vi "choosePlayVSS.vi"(8 "error in (no error)":errorcluster, 10 "queue":T1(array[ring]), 11 "Game in":refnum<class "Game.lvclass">) -> (0 "error out":errorcluster, 2 "output queue":T1(array[ring]), 3 "Game out":refnum<class "Game.lvclass">)   [LabVIEW 2020, in "Game.lvclass"]
uses:
  Game.lvclass
  Command.ctl
  Game.lvclass/Game.ctl
  HaltPlay_class/HaltPlay.lvclass
  TimeoutPlay_class/TimeoutPlay.lvclass
  NormalGamePlayVSS_class/NormalGamePlayVSS.lvclass
  KickPenaltyAllyPlayVSS_class/KickPenaltyAllyPlayVSS.lvclass
  PenaltyEnemyPlayVSS_class/PenaltyEnemyPlayVSS.lvclass
  BallChallengePlayVSS_class/BallChallengePlayVSS.lvclass
  PreparePenaltyAllyPlayVSS_class/PreparePenaltyAllyPlayVSS.lvclass
  DeadBallPlayVSS_class/DeadBallPlayVSS.lvclass
  PreparePenaltyEnemyPlayVSS_class/PreparePenaltyEnemyPlayVSS.lvclass
  PrepareKickoffAllyPlayVSS_class/PrepareKickoffAllyPlayVSS.lvclass
  PrepareKickoffEnemyPlayVSS_class/PrepareKickoffEnemyPlayVSS.lvclass
  StopPlayVSS_class/StopPlayVSS.lvclass
  PrepareGoalKickAllyPlayVSS_class/PrepareGoalKickAllyPlayVSS.lvclass
  PrepareGoalKickEnemyPlayVSS_class/PrepareGoalKickEnemyPlayVSS.lvclass
  KickoffEnemyPlayVSS_class/KickoffEnemyPlayVSS.lvclass
  KickoffAllyPlayVSS_class/KickoffAllyPlayVSS.lvclass
  GoalKickAllyPlayVSS_class/GoalKickAllyPlayVSS.lvclass
  GoalKickEnemyPlayVSS_class/GoalKickEnemyPlayVSS.lvclass
  PrepareFreeBallPlayVSS_class/PrepareFreeBallPlayVSS.lvclass
  FreeBallPlayVSS_class/FreeBallPlayVSS.lvclass
  Read KeeperTeam.vi
  Read Referee.vi
  Read AllyRef.vi
  Write AllyRef.vi
  Write KeeperTeam.vi
  Ally_class/Ally.lvclass
  C:/Users/lucio/Desktop/Horie/ROBOIME/VSS_AI/Team_class/Team.lvclass
  Referee_class/Referee.lvclass
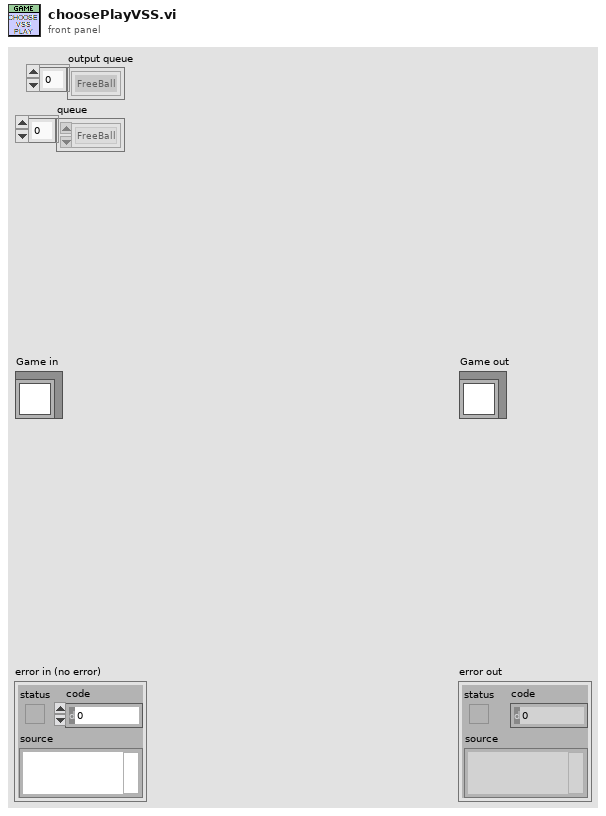
[diagram p1: front panel]
types:
  T1 = enum16{"FreeBall", "PrepareFreeBall", "GoalKickEnemy", "GoalKickAlly", "KickoffAlly", "KickoffEnemy", "PrepareGoalKickEnemy", "PrepareGoalKickAlly", "Stop", "PrepareKickoffEnemy", "PrepareKickoffAlly", "PreparePenaltyEnemy", "Timeout", "DeadBall", "NormalGame", "KickPenaltyAlly", "PenaltyEnemy", "BallChallenge", "PreparePenaltyAlly", "Halt"}[]
  T2 = typedef "Command.ctl" = enum16{"AUTO", "GAME_ON", "STOP", "HALT", "KICKOFF_ALLY", "KICKOFF_ENEMY", "FREE_BALL", "GOAL_KICK_ENEMY", "GOAL_KICK_ALLY", "PENALTY_KICK_ENEMY", "PENALTY_KICK_ALLY", "FREE_KICK"}
  T3 = enum16{"FreeBall", "PrepareFreeBall", "GoalKickEnemy", "GoalKickAlly", "KickoffAlly", "KickoffEnemy", "PrepareGoalKickEnemy", "PrepareGoalKickAlly", "Stop", "PrepareKickoffEnemy", "PrepareKickoffAlly", "PreparePenaltyEnemy", "Timeout", "DeadBall", "NormalGame", "KickPenaltyAlly", "PenaltyEnemy", "BallChallenge", "PreparePenaltyAlly", "Halt"}
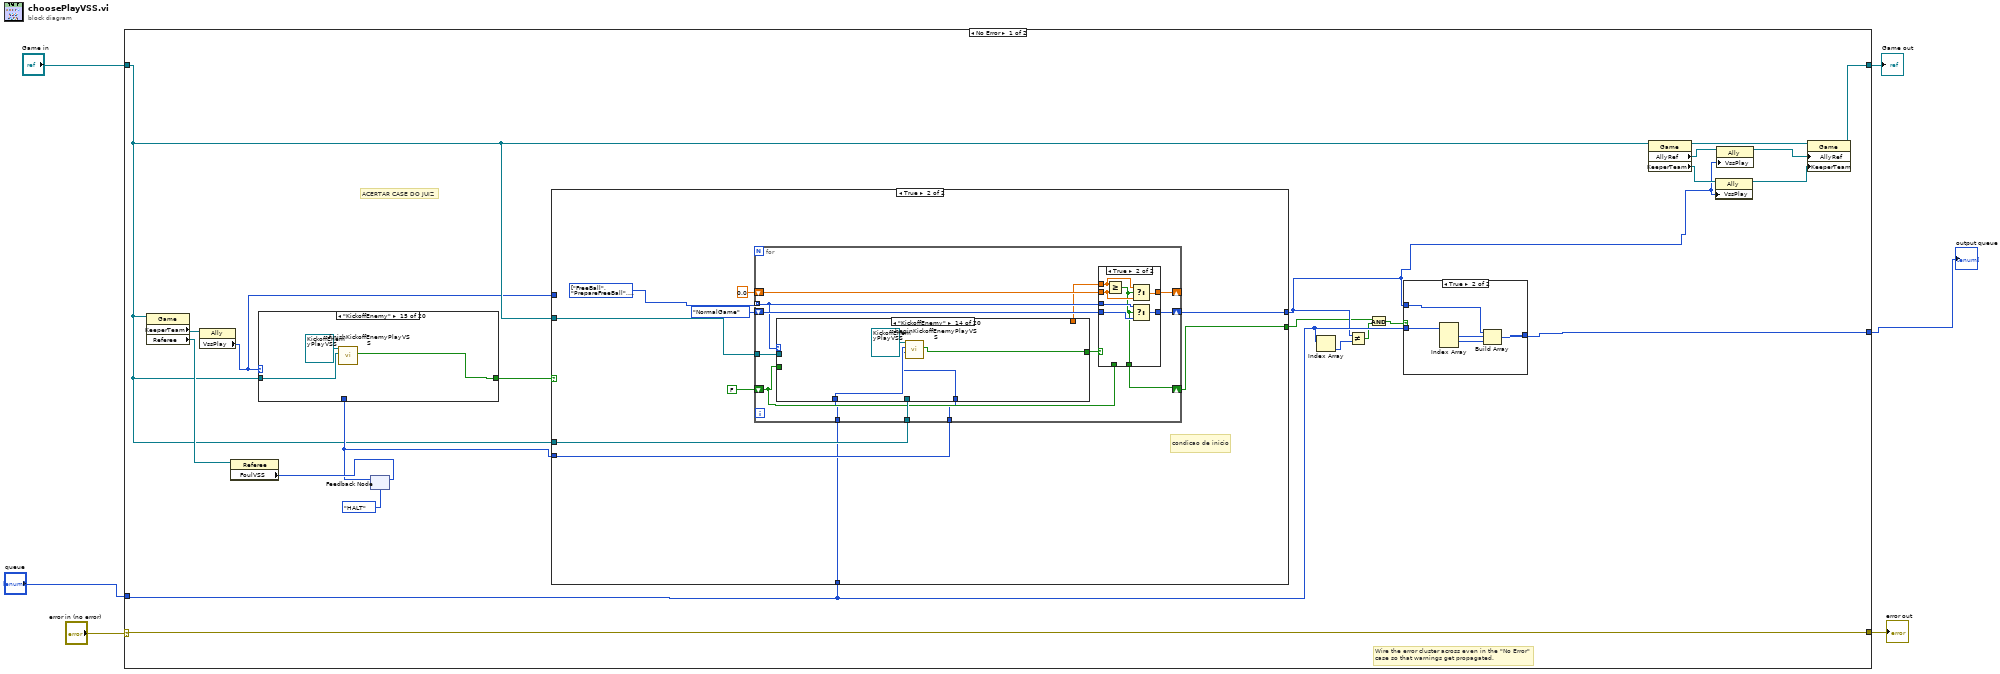
[diagram p0: block diagram]
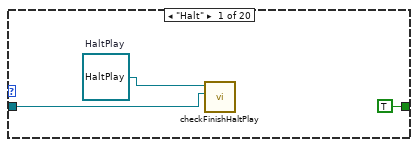
[diagram p3: hidden frame]
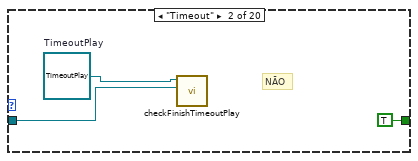
[diagram p4: hidden frame]
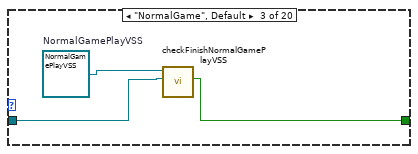
[diagram p5: hidden frame]
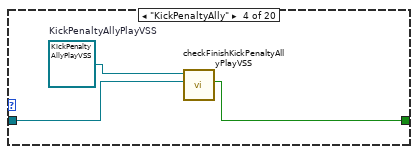
[diagram p6: hidden frame]
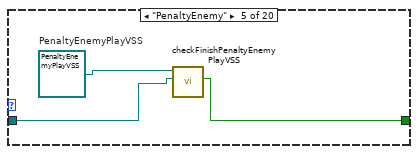
[diagram p7: hidden frame]
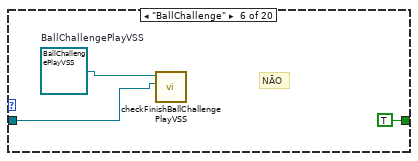
[diagram p8: hidden frame]
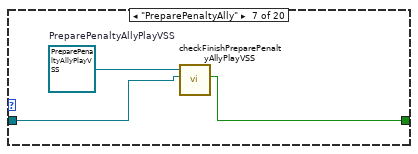
[diagram p9: hidden frame]
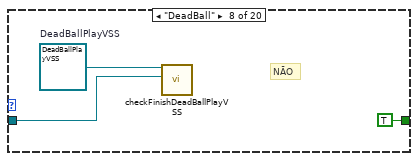
[diagram p10: hidden frame]
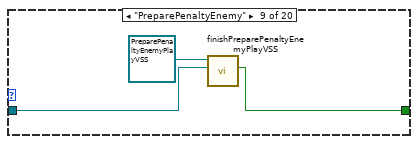
[diagram p11: hidden frame]
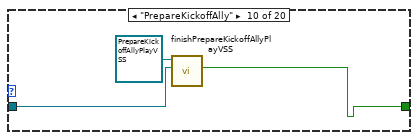
[diagram p12: hidden frame]
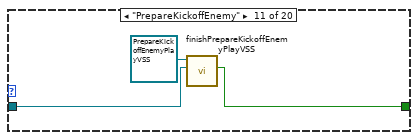
[diagram p13: hidden frame]
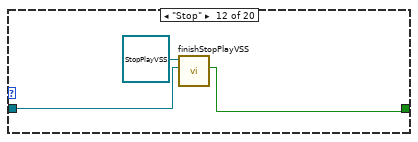
[diagram p14: hidden frame]
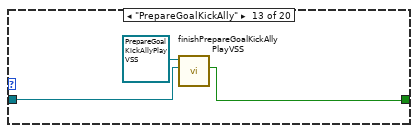
[diagram p15: hidden frame]
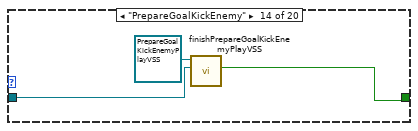
[diagram p16: hidden frame]
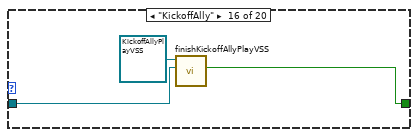
[diagram p17: hidden frame]
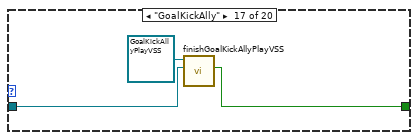
[diagram p18: hidden frame]
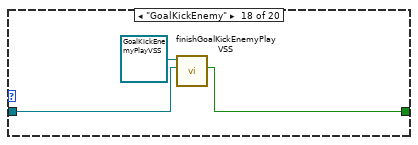
[diagram p19: hidden frame]
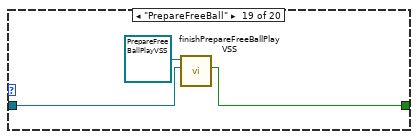
[diagram p20: hidden frame]
diagram:
  n1 = case shown="No Error" "error in (no error)" {
    selector: "error in (no error)" -> [w28 w199]
    tunnel: [w28 w199] -> w5
    tunnel: [w26 w198] -> w3
    tunnel: "Game in" -> [w17 w198]
    tunnel: "queue" -> [w12 _]
    tunnel: [w14 _] -> w1
    frame No Error {
      # "ACERTAR CASE DO JUIZ"
      # "Wire the error cluster across even in the \"No Error\"\ncase so that warnings get propagated."
      n2 = property class="Game"(reference=w17) -> ("KeeperTeam"=w16:refnum<class "Ally.lvclass">, "Referee"=w20:refnum<class "Referee.lvclass">)  [unwired: 1 in, 2 out]
      n3 = property class="Ally"(reference=w16) -> ("VssPlay"=w15:T3)  [unwired: 1 in, 2 out]
      n4 = property class="Referee"(reference=w20) -> ("FoulVSS"=w19:T2)  [unwired: 1 in, 2 out]
      n5 = feedback-in #1(w19) -> ()
      n6 = feedback #1(Command."HALT" ("FoulVSS")) -> (w18:T2)
      n7 = case shown="\"KickoffEnemy\"" w15 {
        tunnel: [TRUE ("result") TRUE ("Boolean") w41 w44 w47 TRUE ("Boolean") w53 TRUE ("Boolean") w59 w62 w65 w68 w71 w74 w77 w80 w83 w86 w89 w92] -> w25
        tunnel: w17 -> [w36 w39 w42 w45 w48 w51 w54 w58 w60 w63 w66 w69 w72 w75 w78 w81 w84 w87 w90 w93]
        tunnel: w18 -> [_ _ _ _ _ _ _ _ _ _ _ _ _ _ _ _ _ _ _ _]
        frame "Halt" {
          w37 = refnum<class "HaltPlay.lvclass"> refnum  # HaltPlay
          n8 = call "checkFinishHaltPlay.vi"("Game"=w36, "HaltPlay in"=w37) -> ()  [unwired: 7 in, 3 out]
        }
        frame "Timeout" {
          w40 = refnum<class "TimeoutPlay.lvclass"> refnum  # TimeoutPlay
          # "NÃO"
          n9 = call "checkFinishTimeoutPlay.vi"("Game"=w39, "TimeoutPlay in"=w40) -> ()  [unwired: 7 in, 3 out]
        }
        frame "NormalGame", Default {
          w43 = refnum<class "NormalGamePlayVSS.lvclass"> refnum  # NormalGamePlayVSS
          n10 = call "checkFinishNormalGamePlayVSS.vi"("Game in"=w42, "NormalGamePlayVSS in"=w43) -> ("Boolean"=w41:bool)  [unwired: 7 in, 2 out]
        }
        frame "KickPenaltyAlly" {
          w46 = refnum<class "KickPenaltyAllyPlayVSS.lvclass"> refnum  # KickPenaltyAllyPlayVSS
          n11 = call "checkFinishKickPenaltyAllyPlayVSS.vi"("Game in"=w45, "KickPenaltyAllyPlayVSS in"=w46) -> ("result"=w44:bool)  [unwired: 7 in, 2 out]
        }
        frame "PenaltyEnemy" {
          w49 = refnum<class "PenaltyEnemyPlayVSS.lvclass"> refnum  # PenaltyEnemyPlayVSS
          n12 = call "checkFinishPenaltyEnemyPlayVSS.vi"("Game in"=w48, "PenaltyEnemyPlayVSS in"=w49) -> ("result"=w47:bool)  [unwired: 7 in, 2 out]
        }
        frame "BallChallenge" {
          w52 = refnum<class "BallChallengePlayVSS.lvclass"> refnum  # BallChallengePlayVSS
          # "NÃO"
          n13 = call "checkFinishBallChallengePlayVSS.vi"("Game in"=w51, "BallChallengePlayVSS in"=w52) -> ()  [unwired: 7 in, 3 out]
        }
        frame "PreparePenaltyAlly" {
          w55 = refnum<class "PreparePenaltyAllyPlayVSS.lvclass"> refnum  # PreparePenaltyAllyPlayVSS
          n14 = call "checkFinishPreparePenaltyAllyPlayVSS.vi"("Game"=w54, "PreparePenaltyAllyPlayVSS in"=w55) -> ("Boolean"=w53:bool)  [unwired: 7 in, 2 out]
        }
        frame "DeadBall" {
          w57 = refnum<class "DeadBallPlayVSS.lvclass"> refnum  # DeadBallPlayVSS
          # "NÃO"
          n15 = call "checkFinishDeadBallPlayVSS.vi"("Game"=w58, "DeadBallPlayVSS in"=w57) -> ()  [unwired: 7 in, 3 out]
        }
        frame "PreparePenaltyEnemy" {
          n16 = call "finishPreparePenaltyEnemyPlayVSS.vi"("Game in"=w60, "PreparePenaltyEnemyPlayVSS in"=refnum<class "PreparePenaltyEnemyPlayVSS.lvclass"> refnum) -> ("Boolean"=w59:bool)  [unwired: 7 in, 2 out]
        }
        frame "PrepareKickoffAlly" {
          n17 = call "finishPrepareKickoffAllyPlayVSS.vi"("Game in"=w63, "PrepareKickoffAllyPlayVSS in"=refnum<class "PrepareKickoffAllyPlayVSS.lvclass"> refnum) -> ("Boolean"=w62:bool)  [unwired: 7 in, 2 out]
        }
        frame "PrepareKickoffEnemy" {
          n18 = call "finishPrepareKickoffEnemyPlayVSS.vi"("Game in"=w66, "PrepareKickoffEnemyPlayVSS in"=refnum<class "PrepareKickoffEnemyPlayVSS.lvclass"> refnum) -> ("Boolean"=w65:bool)  [unwired: 7 in, 2 out]
        }
        frame "Stop" {
          n19 = call "finishStopPlayVSS.vi"("Game in"=w69, "StopPlayVSS in"=refnum<class "StopPlayVSS.lvclass"> refnum) -> ("Boolean"=w68:bool)  [unwired: 7 in, 2 out]
        }
        frame "PrepareGoalKickAlly" {
          n20 = call "finishPrepareGoalKickAllyPlayVSS.vi"("Game in 2"=w72, "PrepareGoalKickAllyPlayVSS in"=refnum<class "PrepareGoalKickAllyPlayVSS.lvclass"> refnum) -> ("Boolean"=w71:bool)  [unwired: 7 in, 2 out]
        }
        frame "PrepareGoalKickEnemy" {
          n21 = call "finishPrepareGoalKickEnemyPlayVSS.vi"("Game in 2"=w75, "PrepareGoalKickEnemyPlayVSS in"=refnum<class "PrepareGoalKickEnemyPlayVSS.lvclass"> refnum) -> ("Boolean"=w74:bool)  [unwired: 7 in, 2 out]
        }
        frame "KickoffEnemy" {
          n22 = call "finishKickoffEnemyPlayVSS.vi"("Game in"=w78, "KickoffEnemyPlayVSS in"=refnum<class "KickoffEnemyPlayVSS.lvclass"> refnum) -> ("result"=w77:bool)  [unwired: 7 in, 2 out]
        }
        frame "KickoffAlly" {
          n23 = call "finishKickoffAllyPlayVSS.vi"("Game in"=w81, "KickoffAllyPlayVSS in"=refnum<class "KickoffAllyPlayVSS.lvclass"> refnum) -> ("result"=w80:bool)  [unwired: 7 in, 2 out]
        }
        frame "GoalKickAlly" {
          n24 = call "finishGoalKickAllyPlayVSS.vi"("Game in"=w84, "GoalKickAllyPlayVSS in"=refnum<class "GoalKickAllyPlayVSS.lvclass"> refnum) -> ("result"=w83:bool)  [unwired: 7 in, 2 out]
        }
        frame "GoalKickEnemy" {
          n25 = call "finishGoalKickEnemyPlayVSS.vi"("Game in"=w87, "GoalKickEnemyPlayVSS in"=refnum<class "GoalKickEnemyPlayVSS.lvclass"> refnum) -> ("result"=w86:bool)  [unwired: 7 in, 2 out]
        }
        frame "PrepareFreeBall" {
          n26 = call "finishPrepareFreeBallPlayVSS.vi"("Game in 2"=w90, "PrepareFreeBallPlayVSS in"=refnum<class "PrepareFreeBallPlayVSS.lvclass"> refnum) -> ("Boolean"=w89:bool)  [unwired: 7 in, 2 out]
        }
        frame "FreeBall" {
          n27 = call "finishFreeBallPlayVSS.vi"("Game in"=w93, "FreeBallPlayVSS in"=refnum<class "FreeBallPlayVSS.lvclass"> refnum) -> ("result"=w92:bool)  [unwired: 7 in, 2 out]
        }
      }
      n28 = case shown="True" w25 {
        tunnel: [w96 w105] -> w10
        tunnel: w15 -> [w96 _]
        tunnel: w17 -> [_ w104]
        tunnel: w18 -> [_ w102]
        tunnel: w17 -> [_ w101]
        tunnel: [FALSE w99] -> w8
        tunnel: w12 -> [_ w98]
        frame False {
        }
        frame True {
          w100 = T1 [enum."FreeBall", enum."PrepareFreeBall", enum."GoalKickEnemy", enum."GoalKickAlly", enum."KickoffAlly", enum."KickoffEnemy", enum."PrepareGoalKickEnemy", enum."PrepareGoalKickAlly", enum."Stop", enum."PrepareKickoffEnemy", enum."PrepareKickoffAlly", enum."PreparePenaltyEnemy", enum."Timeout", enum."DeadBall", enum."KickPenaltyAlly", enum."PenaltyEnemy", enum."BallChallenge", enum."PreparePenaltyAlly", enum."Halt", enum."NormalGame"] items=["FreeBall", "PrepareFreeBall", "GoalKickEnemy", "GoalKickAlly", "KickoffAlly", "KickoffEnemy", "PrepareGoalKickEnemy", "PrepareGoalKickAlly", "Stop", "PrepareKickoffEnemy", "PrepareKickoffAlly", "PreparePenaltyEnemy", "Timeout", "DeadBall", "NormalGame", "KickPenaltyAlly", "PenaltyEnemy", "BallChallenge", "PreparePenaltyAlly", "Halt"] ("VssPlay")
          # "condicao de inicio"
          n29 = for {
            tunnel: w100 -> [w115] mode=indexing
            shift-right: [w118] -> _
            shift-left: 0.0 -> [w117]
            shift-right: [w116] -> w105
            shift-left: T3."NormalGame" ("VssPlay") -> [w119]
            tunnel: w104 -> [w112]
            shift-right: [w111] -> w99
            shift-left: FALSE -> [w110]
            tunnel: w102 -> [w109]
            tunnel: w101 -> [w108]
            tunnel: w98 -> [w107]
            n30 = case shown="\"KickoffEnemy\"" w115 {
              tunnel: [w120 w124 FALSE ("Boolean") w132 FALSE ("Boolean") FALSE ("Boolean") w145 w150 w151 w154 w157 w160 w163 w167 w170 w173 w176 w179 w182 w185] -> w114
              tunnel: [0.0 0.0 0.0 0.0 0.0 0.0 0.0 0.0 _ _ _ _ _ _ _ _ _ _ _ _] -> w113
              tunnel: w112 -> [w122 _ _ _ _ _ _ _ _ w155 _ _ _ _ w171 w175 w177 w180 w183 _]
              tunnel: w110 -> [_ _ _ _ _ _ _ w149 _ _ _ _ _ _ _ _ _ _ _ _]
              tunnel: w109 -> [_ _ _ _ _ _ _ _ _ _ _ _ _ w166 _ _ _ _ _ _]
              tunnel: w108 -> [_ _ w130 _ w137 w141 w146 _ _ _ _ _ _ _ _ _ _ _ _ w186]
              tunnel: w107 -> [_ w125 _ w133 _ _ _ _ w152 _ w158 w161 w164 w168 _ _ _ _ _ _]
              frame "Halt" {
                w123 = refnum<class "HaltPlay.lvclass"> refnum  # HaltPlay
                # "NÃO"
                n31 = call "checkBeginHaltPlay.vi"("Game"=w122, "HaltPlay in"=w123) -> ("Boolean"=w120:bool)  [unwired: 7 in, 2 out]
              }
              frame "KickPenaltyAlly" {
                w126 = refnum<class "KickPenaltyAllyPlayVSS.lvclass"> refnum  # KickPenaltyAllyPlayVSS
                n32 = call "checkBeginKickPenaltyAllyPlayVSS.vi"("queue 2"=w125, "KickPenaltyAllyPlayVSS in"=w126) -> ("logical AND"=w124:bool)  [unwired: 7 in, 2 out]
              }
              frame "Timeout" {
                w131 = refnum<class "TimeoutPlay.lvclass"> refnum  # TimeoutPlay
                # "NÃO"
                n33 = call "checkBeginTimeoutPlay.vi"("Game"=w130, "TimeoutPlay in"=w131) -> ()  [unwired: 7 in, 3 out]
              }
              frame "PenaltyEnemy" {
                n34 = call "checkBeginPenaltyEnemyPlayVSS.vi"("queue 2"=w133, "PenaltyEnemyPlayVSS in"=refnum<class "PenaltyEnemyPlayVSS.lvclass"> refnum) -> ("logical AND"=w132:bool)  [unwired: 7 in, 2 out]
              }
              frame "BallChallenge" {
                # "NÃO"
                n35 = call "checkBeginBallChallengePlayVSS.vi"("Game"=w137, "BallChallengePlayVSS in"=refnum<class "BallChallengePlayVSS.lvclass"> refnum) -> ()  [unwired: 7 in, 3 out]
              }
              frame "DeadBall" {
                # "NÃO"
                n36 = call "checkBeginDeadBallPlayVSS.vi"("Game"=w141, "DeadBallPlayVSS in"=refnum<class "DeadBallPlayVSS.lvclass"> refnum) -> ()  [unwired: 7 in, 3 out]
              }
              frame "PreparePenaltyAlly" {
                w147 = refnum<class "PreparePenaltyAllyPlayVSS.lvclass"> refnum  # PreparePenaltyAllyPlayVSS
                n37 = call "checkBeginPreparePenaltyAllyPlayVSS.vi"("Game in"=w146, "PreparePenaltyAllyPlayVSS in"=w147) -> ("Boolean"=w145:bool)  [unwired: 7 in, 2 out]
              }
              frame "NormalGame", Default {
                n38 = Not(x=w149) -> (.not. x?=w150:bool)
              }
              frame "FreeBall" {
                n39 = call "beginFreeBallPlayVSS.vi"("queue 2"=w152, "FreeBallPlayVSS in"=refnum<class "FreeBallPlayVSS.lvclass"> refnum) -> ("logical AND"=w151:bool)  [unwired: 7 in, 2 out]
              }
              frame "PrepareFreeBall" {
                n40 = call "beginPrepareFreeBallPlayVSS.vi"("Game in"=w155, "PrepareFreeBallPlayVSS in"=refnum<class "PrepareFreeBallPlayVSS.lvclass"> refnum) -> ("Boolean"=w154:bool)  [unwired: 7 in, 2 out]
              }
              frame "GoalKickEnemy" {
                n41 = call "beginGoalKickEnemyPlayVSS.vi"("queue 2"=w158, "GoalKickEnemyPlayVSS in"=refnum<class "GoalKickEnemyPlayVSS.lvclass"> refnum) -> ("logical AND"=w157:bool)  [unwired: 7 in, 2 out]
              }
              frame "GoalKickAlly" {
                n42 = call "beginGoalKickAllyPlayVSS.vi"("queue 2"=w161, "GoalKickAllyPlayVSS in"=refnum<class "GoalKickAllyPlayVSS.lvclass"> refnum) -> ("logical AND"=w160:bool)  [unwired: 7 in, 2 out]
              }
              frame "KickoffAlly" {
                n43 = call "beginKickoffAllyPlayVSS.vi"("queue 2"=w164, "KickoffAllyPlayVSS in"=refnum<class "KickoffAllyPlayVSS.lvclass"> refnum) -> ("logical AND"=w163:bool)  [unwired: 7 in, 2 out]
              }
              frame "KickoffEnemy" {
                n44 = call "beginKickoffEnemyPlayVSS.vi"("FoulVSS"=w166, "queue 2"=w168, "KickoffEnemyPlayVSS in"=refnum<class "KickoffEnemyPlayVSS.lvclass"> refnum) -> ("logical AND"=w167:bool)  [unwired: 6 in, 2 out]
              }
              frame "PrepareGoalKickEnemy" {
                n45 = call "beginPrepareGoalKickEnemyPlayVSS.vi"("Game in"=w171, "PrepareGoalKickEnemyPlayVSS in"=refnum<class "PrepareGoalKickEnemyPlayVSS.lvclass"> refnum) -> ("Boolean"=w170:bool)  [unwired: 7 in, 2 out]
              }
              frame "PrepareGoalKickAlly" {
                n46 = call "beginPrepareGoalKickAllyPlayVSS.vi"("Game in"=w175, "PrepareGoalKickAllyPlayVSS in"=refnum<class "PrepareGoalKickAllyPlayVSS.lvclass"> refnum) -> ("Boolean"=w173:bool)  [unwired: 7 in, 2 out]
              }
              frame "Stop" {
                n47 = call "beginStopPlayVSS.vi"("Game in"=w177, "StopPlayVSS in"=refnum<class "StopPlayVSS.lvclass"> refnum) -> ("Boolean"=w176:bool)  [unwired: 7 in, 2 out]
              }
              frame "PrepareKickoffEnemy" {
                n48 = call "beginPrepareKickoffEnemyPlayVSS.vi"("Game in"=w180, "PrepareKickoffEnemyPlayVSS in"=refnum<class "PrepareKickoffEnemyPlayVSS.lvclass"> refnum) -> ("Boolean"=w179:bool)  [unwired: 7 in, 2 out]
              }
              frame "PrepareKickoffAlly" {
                n49 = call "beginPrepareKickoffAllyPlayVSS.vi"("Game in"=w183, "PrepareKickoffAllyPlayVSS in"=refnum<class "PrepareKickoffAllyPlayVSS.lvclass"> refnum) -> ("Boolean"=w182:bool)  [unwired: 7 in, 2 out]
              }
              frame "PreparePenaltyEnemy" {
                n50 = call "beginPreparePenaltyEnemyPlayVSS.vi"("Game in"=w186, "PreparePenaltyEnemyPlayVSS in"=refnum<class "PreparePenaltyEnemyPlayVSS.lvclass"> refnum) -> ("Boolean"=w185:bool)  [unwired: 7 in, 2 out]
              }
            }
            n51 = case shown="True" w114 {
              tunnel: w119 -> [w189 w194]
              tunnel: [w190 w197] -> w118
              tunnel: w117 -> [w190 w193]
              tunnel: w115 -> [_ w195]
              tunnel: [w189 w196] -> w116
              tunnel: w113 -> [_ w192]
              tunnel: [w188 w191] -> w111
              tunnel: w110 -> [w188 _]
              frame False {
              }
              frame True {
                n52 = Greater Or Equal?(x=w192, y=w193) -> (x >= y?=w191:bool)
                n53 = Select(t=w192, s=w191, f=w193) -> (s? t:f=w197:dbl)
                n54 = Select(t=w195, s=w191, f=w194) -> (s? t:f=w196:T3)
              }
            }
          }
        }
      }
      n55 = Index Array(array=w12) -> (element=w11:T3)  [unwired: 1 in]
      n56 = Not Equal?(x=w10, y=w11) -> (x != y?=w9:bool)
      n57 = And(x=w8, y=w9) -> (x .and. y?=w7:bool)
      n58 = case shown="True" w7 {
        tunnel: w12 -> [w29 w34]
        tunnel: w10 -> [_ w33]
        tunnel: [w29 w30] -> w14
        frame False {
        }
        frame True {
          n59 = Index Array(array=w34) -> (element #1=w32:T3, element #2=w31:T3)  [unwired: 3 in, 1 out]
          n60 = Build Array(w33, w32, w31) -> (w30:T1)
        }
      }
      n61 = property class="Game"(reference=w17) -> (reference out=w27:refnum<class "Game.lvclass">, "AllyRef"=w22:refnum<class "Ally.lvclass">, "KeeperTeam"=w24:refnum<class "Ally.lvclass">)  [unwired: 1 in, 1 out]
      n62 = property class="Ally"(reference=w24, "VssPlay"=w10) -> (reference out=w23:refnum<class "Ally.lvclass">)  [unwired: 1 in, 1 out]
      n63 = property class="Ally"(reference=w22, "VssPlay"=w10) -> (reference out=w21:refnum<class "Ally.lvclass">)  [unwired: 1 in, 1 out]
      n64 = property class="Game"(reference=w27, "AllyRef"=w21, "KeeperTeam"=w23) -> (reference out=w26:refnum<class "Game.lvclass">)  [unwired: 1 in, 1 out]
    }
    frame Error {
    }
  }
  "error out" <- w5
  "Game out" <- w3
  "output queue" <- w1
